vi "StraightenAssociations.vi"(0 "reference":refnum<class "ClassRelationshipEdge.lvclass">, 5 "error in (no error)":errorcluster) -> (14 "reference out":refnum<class "ClassRelationshipEdge.lvclass">, 19 "error out":errorcluster)   [LabVIEW 2014, in "ClassRelationshipEdge.lvclass"]
uses:
  <resource>/Framework/Providers/Open_GDS/UML/ClassRelationshipEdge_class/ClassRelationshipEdge.lvclass
  <resource>/Framework/Providers/Open_GDS/UML/BentStyle_class/BentStyle.lvclass
  <resource>/Framework/Providers/Open_GDS/UML/AbstractNode_class/AbstractNode.lvclass
  <resource>/Framework/Providers/Open_GDS/UML/AbstractEdge_class/AbstractEdge.lvclass
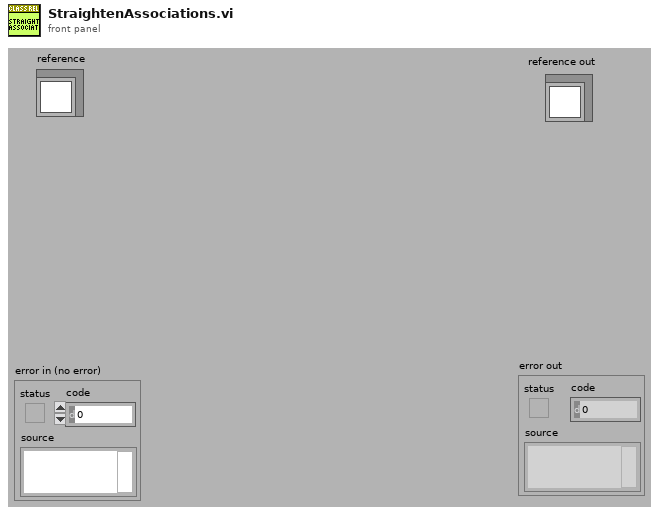
[diagram p1: front panel]
types:
  T1 = typedef "AbstractEdge.lvclass/ObjectAttributes.ctl" = cluster{"start":refnum<class "AbstractNode.lvclass">, "end":refnum<class "AbstractNode.lvclass">}
  T2 = typedef "ClassRelationshipEdge.lvclass/ObjectAttributes.ctl" = cluster{"bentStyleRef":refnum<class "BentStyle.lvclass">, "startConnectionOffset":cluster{"x":i32, "y":i32}, "endConnectionOffset":cluster{"x":i32, "y":i32}, "MidLineOffset":cluster{"x":i32, "y":i32}, "DepClass":T3}
  T3 = typedef "ReversedEngineering_ViDependencyDetailsType.ctl" = cluster{"ThisVIs/Ctls":path[], "Dependent_VIs/Ctls":path[]}
  T4 = typedef "Rectangle Rectangle2D.ctl" = cluster{"x":dbl, "y":dbl, "width":dbl, "height":dbl}
  T5 = typedef "Point Point2D.ctl" = cluster{"x":dbl, "y":dbl}
  T6 = typedef "Direction.lvclass/DirectionTypes.ctl" = enum16{"NORTH", "SOUTH", "EAST", "WEST"}
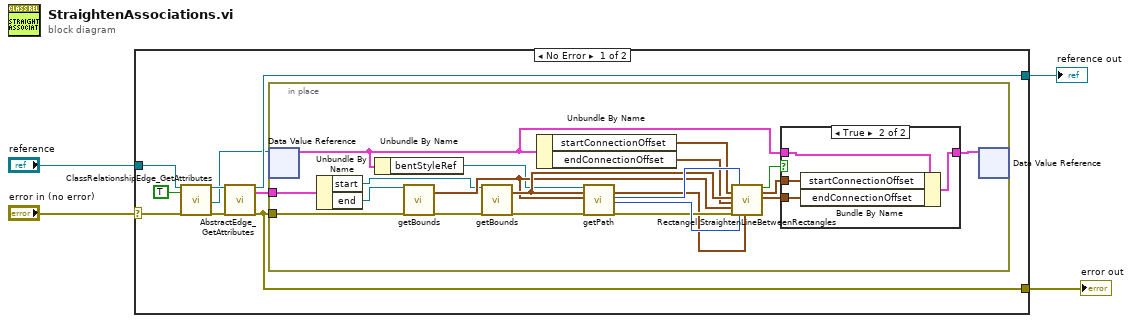
[diagram p0: block diagram]
diagram:
  n1 = case shown="No Error" "error in (no error)" {
    selector: "error in (no error)" -> [w13 w39]
    tunnel: "reference" -> [w12 w40]
    tunnel: [w11 w39] -> w2
    tunnel: [w10 w40] -> w1
    frame No Error {
      n2 = call <resource>:"ClassRelationshipEdge_GetAttributes.vi"("reference in"=w12, "OnlyGetDvrReference(False)"=TRUE, "error in (no error)"=w13) -> ("reference out"=w8:refnum<class "ClassRelationshipEdge.lvclass">, "DataRef"=w5:refnum<data-value>, "error out"=w7:errorcluster)  [unwired: 13 in, 1 out]
      n3 = call <resource>:"AbstractEdge_GetAttributes.vi"("reference in"=w8, "error in (no error)"=w7) -> ("reference out"=w10:refnum<class "ClassRelationshipEdge.lvclass">, "Data"=w6:T1, "error out"=w11:errorcluster)  [unwired: 14 in, 1 out]
      n4 = in-place {
        in-place-border: w11 -> [w33]
        in-place-border: w6 -> [w16]
        n5 = in-place-dvr #1(w5) -> (w15:T2)  [unwired: 1 out]
        n6 = Unbundle By Name(w16) -> ("start"=w18:refnum<class "AbstractNode.lvclass">, "end"=w17:refnum<class "AbstractNode.lvclass">)
        n7 = Unbundle By Name(w15) -> ("bentStyleRef"=w24:refnum<class "BentStyle.lvclass">)
        n8 = call-dynamic "getBounds.vi"("reference"=w17, "error in (no error)"=w33) -> ("bounds"=w26:T4, "error out"=w32:errorcluster)  [unwired: 16 out]
        n9 = call-dynamic "getBounds.vi"("reference"=w18, "error in (no error)"=w32) -> ("bounds"=w27:T4, "error out"=w31:errorcluster)  [unwired: 16 out]
        n10 = Unbundle By Name(w15) -> ("startConnectionOffset"=w23:cluster{"x":i32, "y":i32}, "endConnectionOffset"=w22:cluster{"x":i32, "y":i32})
        n11 = call-dynamic "getPath.vi"("reference"=w24, "start"=w27, "end"=w26, "error in (no error)"=w31) -> ("path"=w25:T5[], "startDirection"=w30:T6, "endDirection"=w29:T6, "error out"=w28:errorcluster)  [unwired: 12 out]
        n12 = call <resource>:"Rectangel StraightenLineBetweenRectangles.vi"("Rect1ConnectionOffset"=w23, "Rect1"=w27, "Rect2ConnectionOffset"=w22, "Rect2"=w26, "error in (no error)"=w28, "Rect1LineDirection"=w30, "Rect2LineDirection"=w29, "path"=w25) -> ("AdjustmentOK"=w21:bool, "Rect1ConnectionOffset"=w20:cluster{"x":i32, "y":i32}, "Rect2ConnectionOffset"=w19:cluster{"x":i32, "y":i32})  [unwired: 9 out]
        n13 = case shown="True" w21 {
          tunnel: [w34 w38] -> w14
          tunnel: w20 -> [_ w37]
          tunnel: w19 -> [_ w36]
          tunnel: w15 -> [w34 w35]
          frame False {
          }
          frame True {
            n14 = Bundle By Name(cluster=w35, "startConnectionOffset"=w37, "endConnectionOffset"=w36) -> (w38:T2)
          }
        }
        n15 = in-place-dvr #1(w14) -> ()  [unwired: 2 out]
      }
    }
    frame Error {
    }
  }
  "reference out" <- w1
  "error out" <- w2
